vi "Configure Downconverter.vi"(0 "VISA resource name":refnum<visa-resource-name>, 5 "Downconverter Fixed LO Frequency (30 GHz)":dbl=30000000000.0 format="%^#_6g", 7 "Downconverter Frequency Context (0: RF)":i32(ring) items=["RF", "IF"], 9 "Downconverter LO Offset (0: Lower Sideband)":i32(ring) items=["Lower Sideband", "Upper Sideband"], 11 "error in (no error)":errorcluster) -> (4 "VISA resource name out":refnum<visa-resource-name>, 15 "error out":errorcluster)   [LabVIEW 2014, in "Agilent ESA PSA Series.lvlib"]
doc: "Configures the downconverter settings if the DUT is a downconverter.\n\n<B>Note:</B> \n\nThis VI is only valid in Noise Figure personality. Use <B>Switch Personality</B> VI to switch to Noise Figure before calling this VI."
uses:
  Agilent ESA PSA Series.lvlib
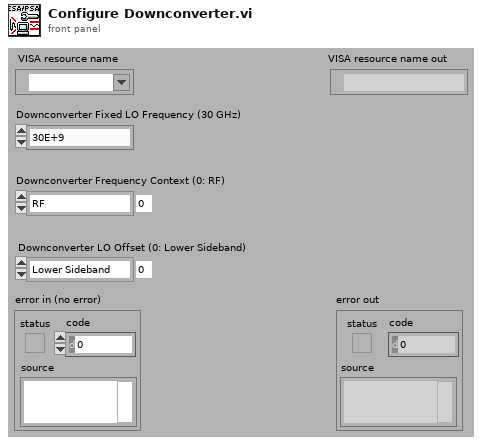
[diagram p1: front panel]
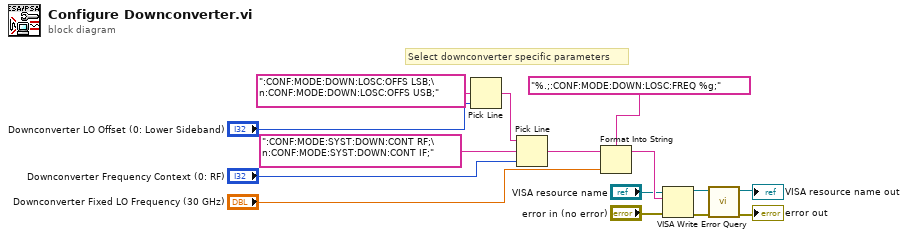
[diagram p0: block diagram]
diagram:
  # "Select downconverter specific parameters"
  n1 = Pick Line(multi-line string=":CONF:MODE:DOWN:LOSC:OFFS LSB;\n:CONF:MODE:DOWN:LOSC:OFFS USB;", line index="Downconverter LO Offset (0: Lower Sideband)") -> (output string=w5:string)  [unwired: 1 in]
  n2 = Pick Line(string ("")=w5, multi-line string=":CONF:MODE:SYST:DOWN:CONT RF;\n:CONF:MODE:SYST:DOWN:CONT IF;", line index="Downconverter Frequency Context (0: RF)") -> (output string=w6:string)
  n3 = Format Into String(format string="%.;:CONF:MODE:DOWN:LOSC:FREQ %g;", initial string=w6, "Downconverter Fixed LO Frequency (30 GHz)") -> (resulting string=w10:string)  [unwired: 1 in, 1 out]
  n4 = VISA Write(VISA resource name="VISA resource name", write buffer=w10, error in (no error)="error in (no error)") -> (VISA resource name out=w13:refnum<visa-resource-name>, error out=w12:errorcluster)  [unwired: 1 out]
  n5 = call "Error Query.vi"("error in (no error)"=w12, "VISA resource name"=w13) -> ("error out"=→"error out":errorcluster, "VISA resource name out"=→"VISA resource name out":refnum<visa-resource-name>)  [unwired: 6 in, 2 out]
